vi "Open TDMS Log File.vi"(7 "TDMS Log File Type":refnum<class "TDMS Log File.lvclass">, 8 "error in (no error)":errorcluster, 9 "Disable Buffering (F)":bool, 10 "Operation":T1, 11 "File Path":path) -> (0 "error out":errorcluster, 3 "TDMS Log File out":refnum<class "TDMS Log File.lvclass">)   [LabVIEW 2015, in "TDMS Log File.lvclass"]
uses:
  TDMS Log File.lvclass
  Log File/Operation.ctl
  Log File/Log File Type.ctl
  Log File/Log File.lvclass/Log File.ctl
  TDMS Log File.lvclass/TDMS Log File.ctl
  Log File/Log File.lvclass
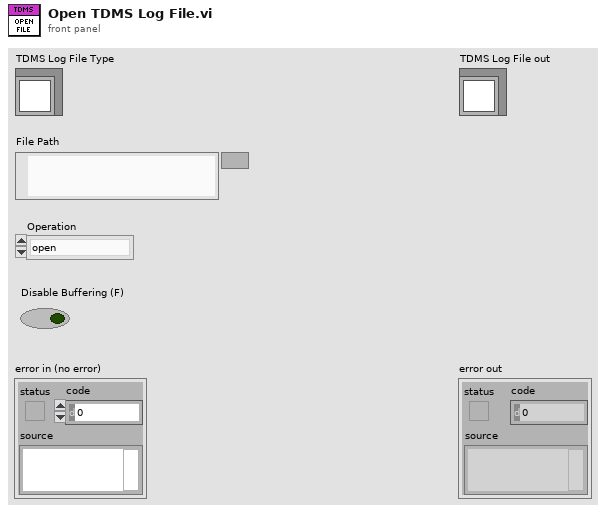
[diagram p1: front panel]
types:
  T1 = typedef "Log File.lvclass/Operation.ctl" = enum16{"open", "open or create", "create or replace", "create", "open (read-only)"}
  T2 = typedef "Log File.lvclass/Log File Type.ctl" = enum16{"Default", "TDMS", "Text"}
  T3 = enum16{"big-endian, network order", "native, host order", "little-endian"}
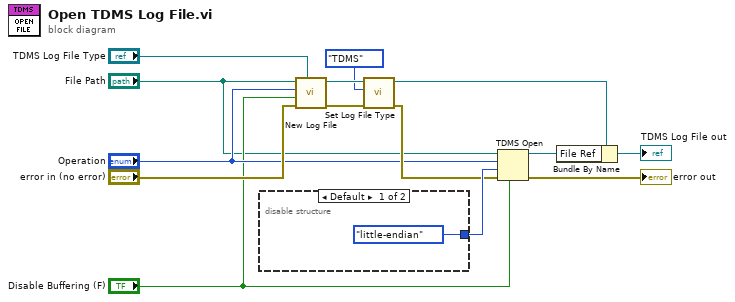
[diagram p0: block diagram]
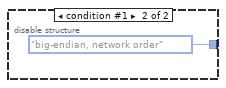
[diagram p2: hidden frame]
diagram:
  n1 = disable-structure shown="Default" {
    disable-tunnel: [T3."little-endian" ("byte order (2:little-endian)") T3."big-endian, network order" ("byte order (2:little-endian)")] -> w10
    frame condition #0 (active) {
    }
    frame condition #1 {
    }
  }
  n2 = call "New Log File.vi"("Log File Type"="TDMS Log File Type", "error in (no error)"="error in (no error)", "Disable Buffering (F)"="Disable Buffering (F)", "Operation"="Operation", "File Path"="File Path") -> ("error out"=w9:errorcluster, "Log File out"=w8:refnum<class "TDMS Log File.lvclass">)  [unwired: 5 in]
  n3 = call "Set Log File Type.vi"("error in (no error)"=w9, "Log File Type"=Log_File_Type."TDMS", "Log File in"=w8) -> ("error out"=w4:errorcluster, "Log File out"=w7:refnum<class "TDMS Log File.lvclass">)  [unwired: 7 in]
  n4 = TDMS Open(6:"Disable Buffering (F)", 8:w4, 9:w10, 10:"Operation", 11:"File Path") -> (0:→"error out":errorcluster, 3:w13:refnum<k34>)  [unwired: 2 in]
  n5 = Bundle By Name(cluster=w7, "File Ref"=w13) -> (→"TDMS Log File out":refnum<class "TDMS Log File.lvclass">)
